vi "PRIOR_IFilterHome.vi"(8 "error in (no error)":errorcluster, 10 "Filter Wheel #":i32=1, 11 "PRIORLib In":T1) -> (0 "error out":errorcluster, 2 "Return":i32, 3 "PRIORLib Out":T1)   [LabVIEW 2009]
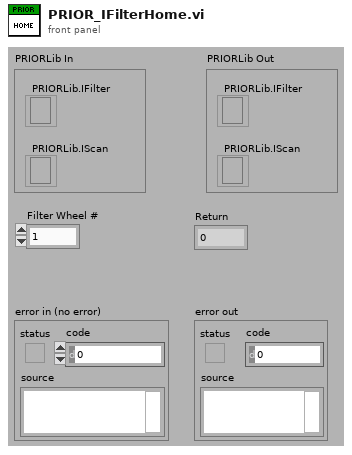
[diagram p1: front panel]
types:
  T1 = cluster{"PRIORLib.IFilter":refnum<k7>, "PRIORLib.IScan":refnum<k7>}
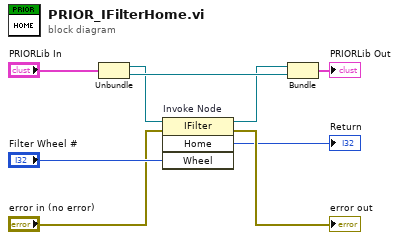
[diagram p0: block diagram]
diagram:
  n1 = Unbundle("PRIORLib In") -> ("PRIORLib.IFilter"=w1:refnum<k7>, "PRIORLib.IScan"=w4:refnum<k7>)
  n2 = invoke on="Invoke Node" class="IFilter" method="Home"(reference=w1, error in="error in (no error)", "Wheel"="Filter Wheel #") -> (reference out=w2:refnum<k7>, error out=→"error out":errorcluster, "Home"=→"Return":i32)  [unwired: 1 in, 1 out]
  n3 = Bundle("PRIORLib.IFilter"=w2, "PRIORLib.IScan"=w4) -> (→"PRIORLib Out":T1)  [unwired: 1 in]
